vi "Retrieve RPC Response.vi"(11 "RPC Response":T1) -> (3 "Output":string[][](array[string]))   [LabVIEW 2017]
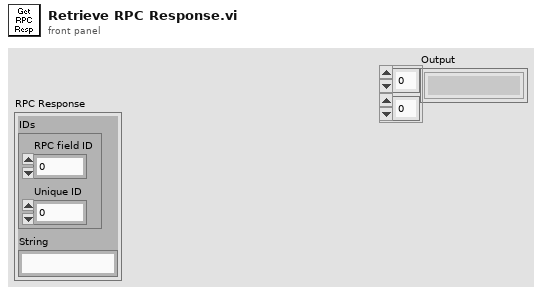
[diagram p1: front panel]
types:
  T1 = cluster{"IDs":cluster{"RPC field ID":u16, "Unique ID":u16}, "String":string}
  T2 = typedef "Field Data.ctl" = cluster{"Dbl":dbl, "String":string, "Type":T3, "Boolean":bool, "Sequence #":T4, "Flags":u8}
  T3 = typedef "Field Type.ctl" = enum8{"Invalid", "Bool", "Numeric", "String", "Raw", "Boolean Array", "Numeric Array", "String Array", "RPC"}
  T4 = typedef "Sequence.ctl" = u16
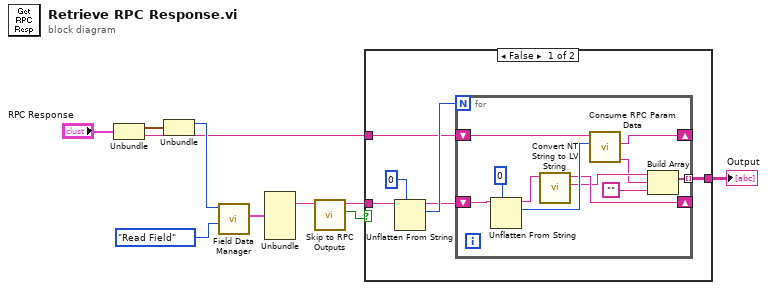
[diagram p0: block diagram]
diagram:
  n1 = Unbundle("RPC Response") -> ("IDs"=w3:cluster{"RPC field ID":u16, "Unique ID":u16}, "String"=w2:string)
  n2 = Unbundle(w3) -> ("RPC field ID"=w9:u16)  [unwired: 1 out]
  n3 = call <vilib>:"Field Data Manager.vi"("Operation"=enum16{"Update Field", "Read Field"}."Read Field", "Field ID"=w9) -> ("Field Value Out"=w8:T2)  [unwired: 8 in, 1 out]
  n4 = Unbundle(w8) -> ("String"=w7:string)  [unwired: 5 out]
  n5 = call <vilib>:"Skip to RPC Outputs.vi"("String in"=w7) -> ("Aborted"=w5:bool, "String out"=w6:string)  [unwired: 8 in, 1 out]
  n6 = case shown="False" w5 {
    tunnel: w6 -> [w15 _]
    tunnel: w2 -> [w12 _]
    tunnel: [w11 _] -> w1
    frame False {
      n7 = Unflatten From String(type=u8 0 ("bytes to read"), binary string=w15) -> (rest of the binary string=w13:string, value=w14:u8)  [unwired: 3 in, 1 out]
      n8 = for {
        N: w14 -> [_]
        shift-right: [w21] -> _
        shift-left: w12 -> [w23]
        shift-right: [w22] -> _
        shift-left: w13 -> [w25]
        tunnel: [w19] -> w11 mode=indexing
        n9 = Unflatten From String(type=u8 0 ("bytes to read"), binary string=w25) -> (rest of the binary string=w26:string, value=w24:u8)  [unwired: 3 in, 1 out]
        n10 = call <vilib>:"Convert NT String to LV String.vi"("Buffer in"=w26) -> ("String Contents"=w20:string, "Remaining String"=w22:string)  [unwired: 8 in, 1 out]
        n11 = call <vilib>:"Consume RPC Param Data.vi"("type"=w24, "RPC String in"=w23) -> ("Value String"=w18:string, "string out"=w21:string)  [unwired: 6 in, 2 out]
        n12 = Build Array(w20, w18, "") -> (w19:string[])
      }
    }
    frame True {
    }
  }
  "Output" <- w1
